vi "CalcTemp.vi"(8 "error in":errorcluster, 11 "ArrayIn":u8[](array[numeric])) -> (0 "error out":errorcluster, 2 "Temp":dbl, 3 "TempRounded":dbl)   [LabVIEW 2014, in "Temp_AS6200.lvlib"]
uses:
  Temp_AS6200.lvlib
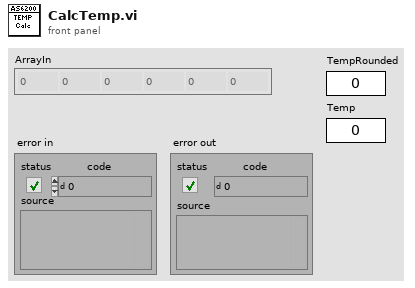
[diagram p1: front panel]
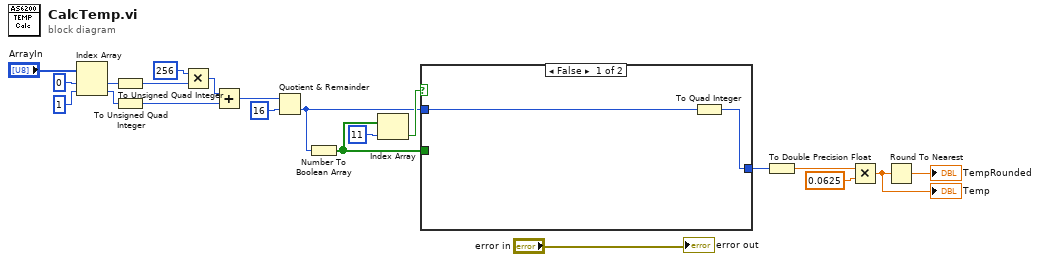
[diagram p0: block diagram]
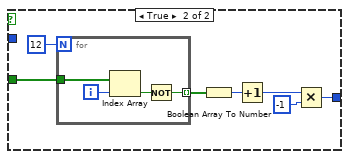
[diagram p2: hidden frame]
diagram:
  n1 = Index Array(array="ArrayIn", index #1=0 ("index"), index #2=1 ("index")) -> (element #1=w7:u8, element #2=w8:u8)
  n2 = To Unsigned Quad Integer(1:w7) -> (0:w9:u64)
  n3 = To Unsigned Quad Integer(1:w8) -> (0:w12:u64)
  n4 = Multiply(x=u64 256, y=w9) -> (x*y=w11:u64)
  n5 = Add(x=w11, y=w12) -> (x+y=w13:u64)
  n6 = Quotient & Remainder(x=w13, y=u64 16) -> (floor(x/y)=w4:u64)  [unwired: 1 out]
  n7 = Number To Boolean Array(number=w4) -> (Boolean array=w17:bool[])
  n8 = Index Array(array=w17, index=11) -> (element=w16:bool)
  n9 = case shown="False" w16 {
    tunnel: w17 -> [_ w30]
    tunnel: [w23 w24] -> w18
    tunnel: w4 -> [w22 _]
    frame False {
      n10 = To Quad Integer(1:w22) -> (0:w23:i64)
    }
    frame True {
      n11 = for {
        N: 12 -> [_]
        tunnel: w30 -> [w34]
        tunnel: [w31] -> w28 mode=indexing
        i -> [w33]
        n12 = Index Array(array=w34, index=w33) -> (element=w32:bool)
        n13 = Not(x=w32) -> (.not. x?=w31:bool)
      }
      n14 = Boolean Array To Number(Boolean array=w28) -> (number=w27:u32)
      n15 = Increment(x=w27) -> (x+1=w26:u32)
      n16 = Multiply(x=w26, y=-1) -> (x*y=w24:u32)
    }
  }
  n17 = To Double Precision Float(number=w18) -> (double precision float=w19:dbl)
  n18 = Multiply(x=w19, y=0.0625) -> (x*y=w2:dbl)
  "Temp" <- w2
  n19 = Round To Nearest(number=w2) -> (nearest integer value=→"TempRounded":dbl)
  "error out" <- "error in"
